vi "_Destroy.vi"(8 "error in (no error)":errorcluster, 11 "StopSignal":T1) -> (0 "error out":errorcluster)   [LabVIEW 2017, in "StopSignal.lvlib"]
uses:
  StopSignal.lvlib
  Typedef/StopSignal.ctl
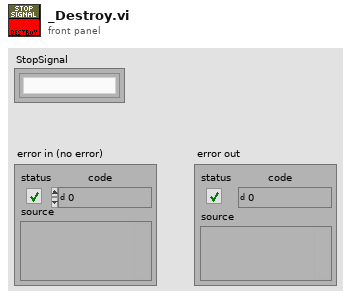
[diagram p1: front panel]
types:
  T1 = typedef "StopSignal.lvlib/StopSignal.ctl" = refnum<k1>
  T2 = typedef "StopSignal.lvlib/Def-StopSignalData.ctl" = cluster{"StopEvent":refnum<user-event>, "StopNotifier":refnum<notifier>, "StopReason":T3}
  T3 = typedef "StopSignal.lvlib/def-StopReason.ctl" = cluster{"Reason":string, "timestamp":timestamp}
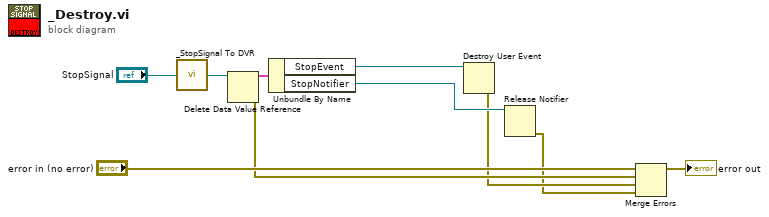
[diagram p0: block diagram]
diagram:
  n1 = call "_StopSignal To DVR.vi"("Refnum in"="StopSignal") -> ("Data Value Reference out"=w9:refnum<data-value>)
  n2 = Delete Data Value Reference(data value reference=w9) -> (data value=w8:T2, error out=w3:errorcluster)  [unwired: 1 in]
  n3 = Unbundle By Name(w8) -> ("StopEvent"=w7:refnum<user-event>, "StopNotifier"=w6:refnum<notifier>)
  n4 = Destroy User Event(user event=w7) -> (error out=w2:errorcluster)  [unwired: 1 in]
  n5 = Release Notifier(notifier=w6) -> (error out=w1:errorcluster)  [unwired: 2 in, 2 out]
  n6 = Merge Errors("error in (no error)", w3, w2, w1) -> (→"error out":errorcluster)
